vi "高速脉冲脚本.vi"(8 "4-wire":bool, 11 "波形":waveform(dbl)) -> (3 "Script":string)   [LabVIEW 2020, in "功能选择.xctl"]
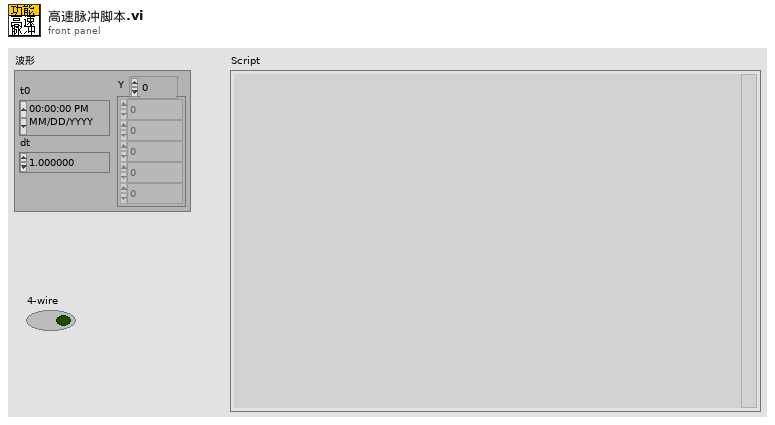
[diagram p1: front panel]
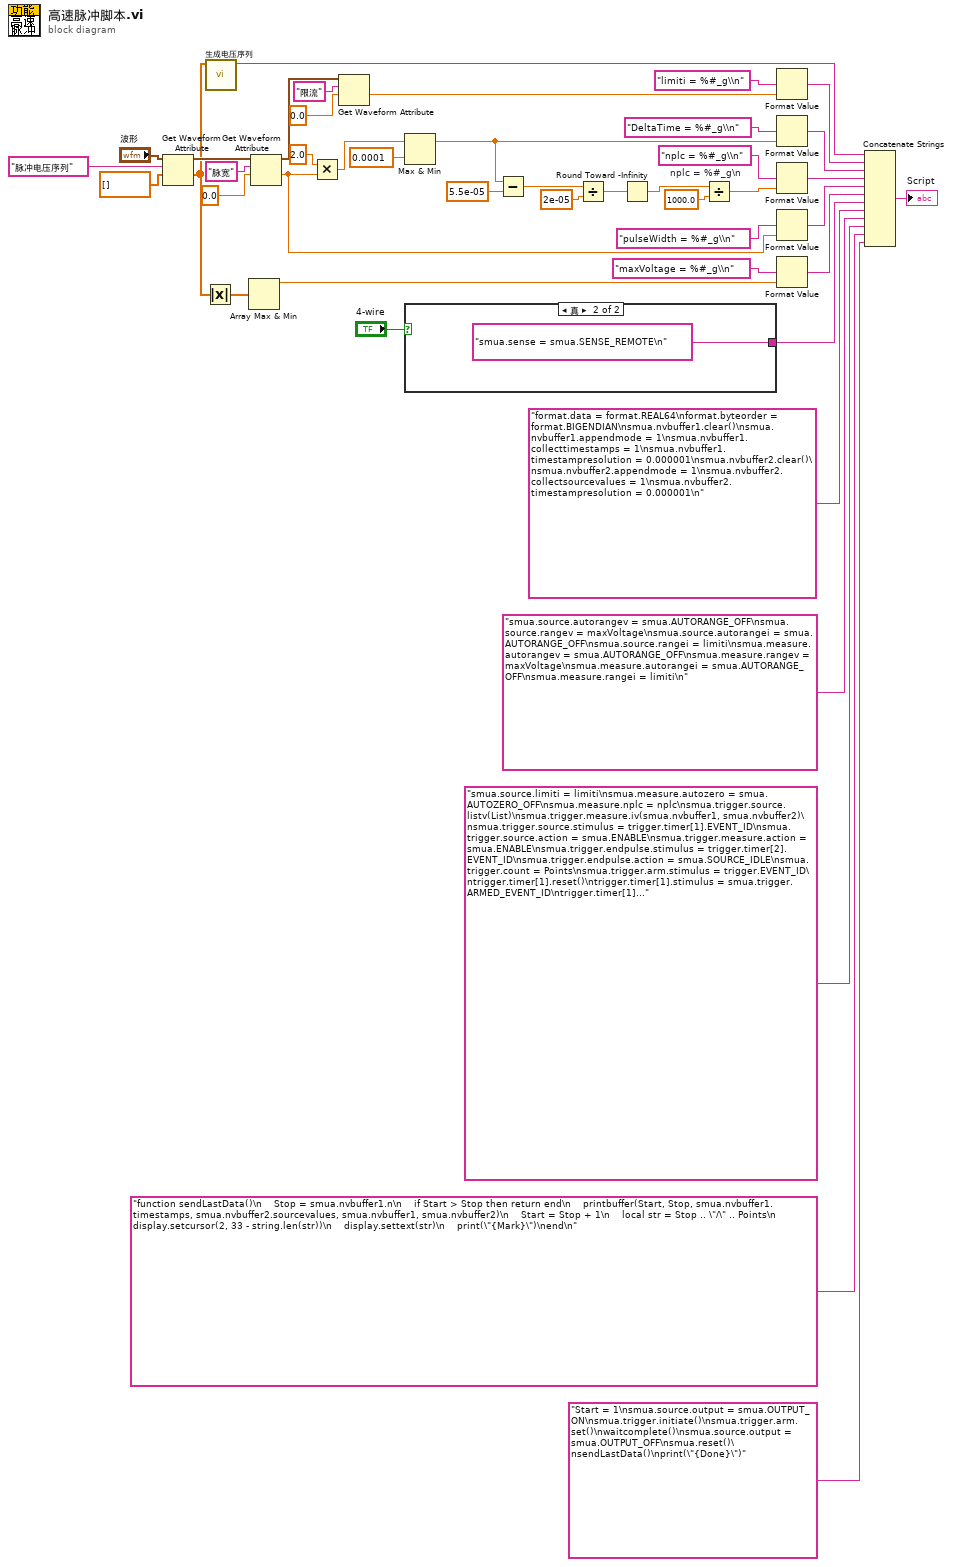
[diagram p0: block diagram]
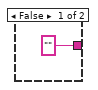
[diagram p2: hidden frame]
diagram:
  w27 = "nplc = %#_g\\n"  # nplc = %#_g\n
  n1 = Get Waveform Attribute(5:dbl[] [], 6:"脉冲电压序列" ("名称"), 7:"波形") -> (1:w28:dbl[], 3:w36:waveform(dbl))  [unwired: 1 in, 2 out]
  n2 = Absolute Value(x=w28) -> (abs(x)=w1:dbl[])
  n3 = call "生成电压序列.vi"("电压序列"=w28) -> ("List"=w17:string)  [unwired: 10 in]
  n4 = Array Max & Min(array=w1) -> (max value=w29:dbl)  [unwired: 3 out]
  n5 = Get Waveform Attribute(5:0.0, 6:"脉宽" ("名称"), 7:w36) -> (1:w24:dbl, 3:w16:waveform(dbl))  [unwired: 1 in, 2 out]
  n6 = Multiply(x=2.0, y=w24) -> (x*y=w32:dbl)
  n7 = Get Waveform Attribute(5:0.0, 6:"限流" ("名称"), 7:w16) -> (1:w13:dbl)  [unwired: 1 in, 3 out]
  n8 = Max & Min(x=w32, y=0.0001) -> (max(x,y)=w3:dbl)  [unwired: 1 out]
  n9 = case shown="真" "4-wire" {
    tunnel: ["" "smua.sense = smua.SENSE_REMOTE\n"] -> w12
    frame False {
    }
    frame True {
    }
  }
  n10 = Subtract(x=w3, y=5.5e-05) -> (x-y=w6:dbl)
  n11 = Divide(x=w6, y=2e-05 ("x")) -> (x/y=w9:dbl)
  n12 = Round Toward -Infinity(1:w9) -> (0:w4:dbl)
  n13 = Divide(x=w4, y=1000.0) -> (x/y=w2:dbl)
  n14 = Format Value(format string="limiti = %#_g\\n" ("格式字符串"), value (0)=w13) -> (output string=w22:string)  [unwired: 1 in]
  n15 = Format Value(format string="DeltaTime = %#_g\\n" ("格式字符串"), value (0)=w3) -> (output string=w21:string)  [unwired: 1 in]
  n16 = Format Value(format string=w27, value (0)=w2) -> (output string=w20:string)  [unwired: 1 in]
  n17 = Format Value(format string="pulseWidth = %#_g\\n" ("格式字符串"), value (0)=w24) -> (output string=w19:string)  [unwired: 1 in]
  n18 = Format Value(format string="maxVoltage = %#_g\\n" ("格式字符串"), value (0)=w29) -> (output string=w18:string)  [unwired: 1 in]
  n19 = Concatenate Strings(w17, w22, w21, w20, w19, w18, w12, "format.data = format.REAL64\nformat.byteorder = format.BIGENDIAN\nsmua.nvbuffer1.clear()\nsmua.nvbuffer1.appendmode = 1\nsmua.nvbuffer1.collecttimestamps = 1\nsmua.nvbuffer1.timestampresolution = 0.000001\nsmua.nvbuffer2.clear()\nsmua.nvbuffer2.appendmode = 1\nsmua.nvbuffer2.collectsourcevalues = 1\nsmua.nvbuffer2.timestampresolution = 0.000001\n", "smua.source.autorangev = smua.AUTORANGE_OFF\nsmua.source.rangev = maxVoltage\nsmua.source.autorangei = smua.AUTORANGE_OFF\nsmua.source.rangei = limiti\nsmua.measure.autorangev = smua.AUTORANGE_OFF\nsmua.measure.rangev = maxVoltage\nsmua.measure.autorangei = smua.AUTORANGE_OFF\nsmua.measure.rangei = limiti\n", "smua.source.limiti = limiti\nsmua.measure.autozero = smua.AUTOZERO_OFF\nsmua.measure.nplc = nplc\nsmua.trigger.source.listv(List)\nsmua.trigger.measure.iv(smua.nvbuffer1, smua.nvbuffer2)\nsmua.trigger.source.stimulus = trigger.timer[1].EVENT_ID\nsmua.trigger.source.action = smua.ENABLE\nsmua.trigger.measure.action = smua.ENABLE\nsmua.trigger.endpulse.stimulus = trigger.timer[2].EVENT_ID\nsmua.trigger.endpulse.action = smua.SOURCE_IDLE\nsmua.trigger.count = Points\nsmua.trigger.arm.stimulus = trigger.EVENT_ID\ntrigger.timer[1].reset()\ntrigger.timer[1].stimulus = smua.trigger.ARMED_EVENT_ID\ntrigger.timer[1].passthrough = false\ntrigger.timer[1].delay = DeltaTime\ntrigger.timer[1].count = Points\ntrigger.timer[2].reset()\ntrigger.timer[2].stimulus = trigger.timer[1].EVENT_ID\ntrigger.timer[2].passthrough = false\ntrigger.timer[2].delay = pulseWidth\ntrigger.timer[2].count = 1\n" ("字符串"), "function sendLastData()\n    Stop = smua.nvbuffer1.n\n    if Start > Stop then return end\n    printbuffer(Start, Stop, smua.nvbuffer1.timestamps, smua.nvbuffer2.sourcevalues, smua.nvbuffer1, smua.nvbuffer2)\n    Start = Stop + 1\n    local str = Stop .. \"/\" .. Points\n    display.setcursor(2, 33 - string.len(str))\n    display.settext(str)\n    print(\"{Mark}\")\nend\n", "Start = 1\nsmua.source.output = smua.OUTPUT_ON\nsmua.trigger.initiate()\nsmua.trigger.arm.set()\nwaitcomplete()\nsmua.source.output = smua.OUTPUT_OFF\nsmua.reset()\nsendLastData()\nprint(\"{Done}\")" ("字符串")) -> (→"Script":string)
